vi "HGF_SVVarManVisitor_create.appendData2Variant.vi"(0 "variant":variant, 2 "SV Name":string, 3 "return-to Event":refnum<class "HGF_TriggeredEvent.lvclass">, 5 "error in":errorcluster) -> (14 "dup variant":variant, 19 "error out":errorcluster)   [LabVIEW 2012, in "HGF_SV.lvlib" / "HGF_SVVarManVisitor_create.lvclass"]
uses:
  HGF_SVVarManVisitor_create.lvclass
  HGF_BaseClasses/HGF_TriggeredEvent/HGF_TriggeredEvent.lvclass
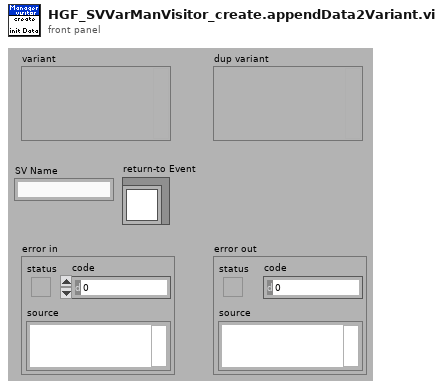
[diagram p1: front panel]
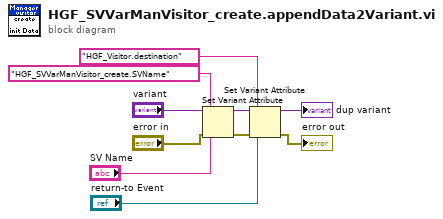
[diagram p0: block diagram]
diagram:
  n1 = Set Variant Attribute(Variant="variant", name="HGF_SVVarManVisitor_create.SVName", value="SV Name", error in="error in") -> (Variant out=w7:variant, error out=w5:errorcluster)  [unwired: 1 out]
  n2 = Set Variant Attribute(Variant=w7, name="HGF_Visitor.destination", value="return-to Event", error in=w5) -> (Variant out=→"dup variant":variant, error out=→"error out":errorcluster)  [unwired: 1 out]
